vi "Global.vi"() -> ()   [LabVIEW 2019]
panel:
  out "bos":bool
  out "spill_id":i64
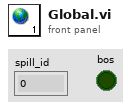
[diagram p1: front panel]
diagram:
